vi "FPGA Write Array By Name - U64.vi"(8 "error in (no error)":errorcluster, 9 "Array":u64[](array[numeric]), 10 "Control":string, 11 "FPGA Session In":refnum<class "FPGA Interface Base.lvclass">) -> (0 "error out":errorcluster, 3 "FPGA Session Out":refnum<class "FPGA Interface Base.lvclass">)   [LabVIEW 2010, in "FPGA Interface Base.lvclass"]
doc: "Writes an entire array of unsigned 64-bit integer values to a given array control or indicator."
uses:
  <userlib>/_FPGA Interface Advanced Tools/FPGA Interface Base/FPGA Interface Base.lvclass
  <vilib>/rvi/DataTransferAndStorage/Container/Common/niFpgaDataTypeControl.ctl
  <userlib>/_FPGA Interface Advanced Tools/FPGA Interface Base/FPGA Interface Base.lvclass/FPGA Interface Base.ctl
  <userlib>/_FPGA Interface Advanced Tools/FPGA Interface Base/Accessors/FPGA Read Session.vi
  <userlib>/_FPGA Interface Advanced Tools/FPGA Interface Wrapper/FPGA Interface Wrapper.lvlib
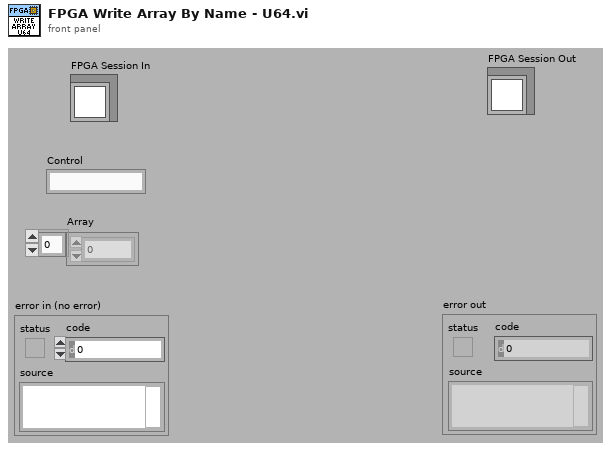
[diagram p1: front panel]
types:
  T1 = typedef "niFpgaDataTypeControl.ctl" = enum32{"Boolean", "I8", "I16", "I32", "I64", "U8", "U16", "U32", "U64", "FXP", "CustomControl"}
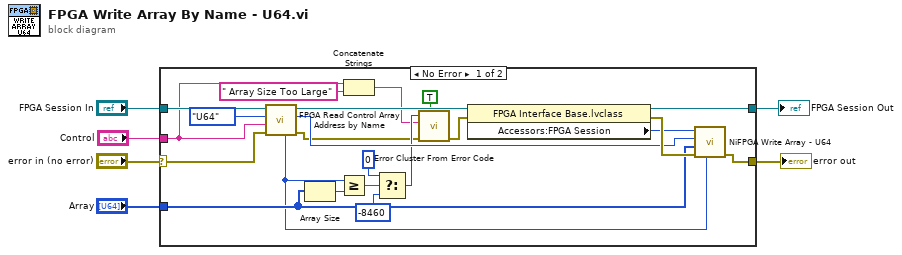
[diagram p0: block diagram]
diagram:
  n1 = case shown="No Error" "error in (no error)" {
    selector: "error in (no error)" -> [w24 w30]
    tunnel: [w25 w30] -> w1
    tunnel: [w26 w29] -> w2
    tunnel: "FPGA Session In" -> [w22 w29]
    tunnel: "Control" -> [w7 _]
    tunnel: "Array" -> [w19 _]
    frame No Error {
      n2 = call <userlib>:"FPGA Read Control Array Address by Name.vi"("error in (no error)"=w24, "Name"=w7, "Data Type"=niFpgaDataTypeControl."U64", "FPGA Interface Base in"=w22) -> ("error out"=w9:errorcluster, "Address"=w20:u32, "FPGA Interface Base out"=w21:refnum<class "FPGA Interface Base.lvclass">, "Num Elements"=w17:u32)  [unwired: 3 in, 1 out]
      n3 = Array Size(array=w19) -> (size(s)=w18:i32)
      n4 = Greater Or Equal?(x=w17, y=w18) -> (x >= y?=w10:bool)
      n5 = Concatenate Strings(w7, " Array Size Too Large" ("string")) -> (w11:string)
      n6 = Select(t=0, s=w10, f=-8460 ("error code (0)")) -> (s? t:f=w16:i32)
      n7 = call <vilib>:"Error Cluster From Error Code.vi"("show call chain? (False)"=TRUE, "error in (no error)"=w9, "error message (\"\")"=w11, "error code (0)"=w16) -> ("error out"=w8:errorcluster)  [unwired: 5 in]
      n8 = property class="FPGA Interface Base.lvclass"(reference=w21, error in=w8) -> (reference out=w26:refnum<class "FPGA Interface Base.lvclass">, error out=w28:errorcluster, "Accessors:FPGA Session"=w27:u32)
      n9 = call <userlib>:"NiFPGA Write Array - U64.vi"("Size"=w17, "error in (no error)"=w28, "Array"=w19, "Control"=w20, "Session"=w27) -> ("error out"=w25:errorcluster)  [unwired: 5 in, 1 out]
    }
    frame Error {
    }
  }
  "error out" <- w1
  "FPGA Session Out" <- w2
